vi "UDP Send.vi"(2 "Selected Target Info":T1, 3 "connection ID":refnum<k16>, 4 "port":u16) -> (5 "connection ID out":refnum<k16>)   [LabVIEW 2011]
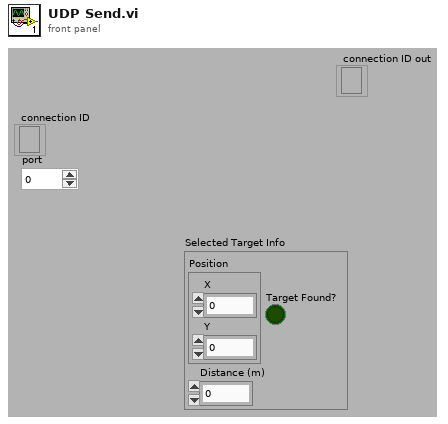
[diagram p1: front panel]
types:
  T1 = cluster{"Position":cluster{"X":dbl, "Y":dbl}, "Distance (m)":dbl, "Target Found?":bool}
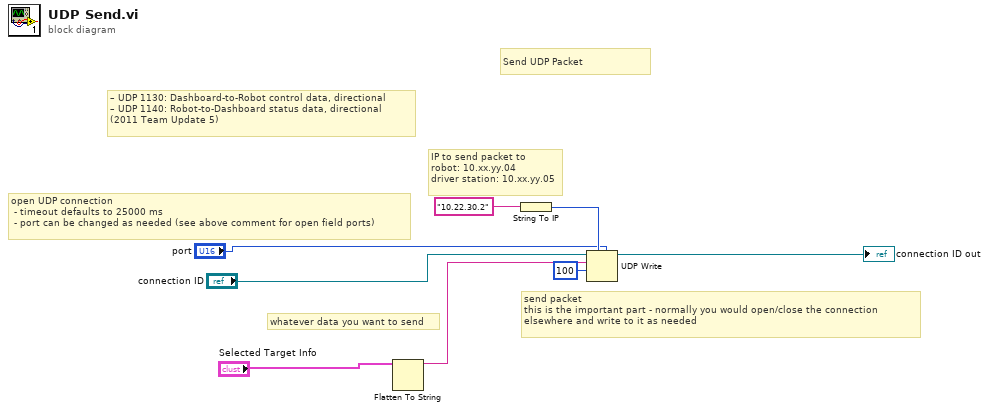
[diagram p0: block diagram]
diagram:
  # "send packet\nthis is the important part - normally you would open/close the connection \nelsewhere and write to it as needed"
  # "whatever data you want to send"
  # "IP to send packet to \nrobot: 10.xx.yy.04\ndriver station: 10.xx.yy.05"
  # "open UDP connection\n - timeout defaults to 25000 ms\n - port can be changed as needed (see above comment for open field ports)"
  # "Send UDP Packet"
  # "– UDP 1130: Dashboard-to-Robot control data, directional\n– UDP 1140: Robot-to-Dashboard status data, directional\n(2011 Team Update 5)"
  n1 = Flatten To String(anything="Selected Target Info") -> (data string=w6:string)  [unwired: 1 in, 4 out]
  n2 = String To IP(1:"10.22.30.2") -> (0:w7:u32)
  n3 = UDP Write(address=w7, port or service name="port", connection ID="connection ID", data in=w6, 9:100 ("timeout ms (25000)")) -> (3:→"connection ID out":refnum<k16>)  [unwired: 1 in, 1 out]
